vi "FitsCloseFile.vi"(8 "error in (no error)":errorcluster, 10 "ref in":u64, 11 "CFitsIO in":refnum<class "CFitsIO.lvclass">) -> (0 "error out":errorcluster, 1 "result":i32, 2 "ref out":u64, 3 "CFitsIO out":refnum<class "CFitsIO.lvclass">)   [LabVIEW 2016, in "CFitsIO.lvclass"]
uses:
  CFitsIO.lvclass
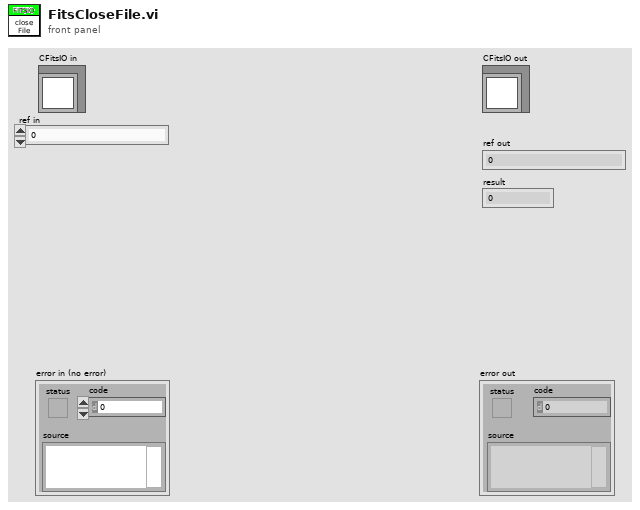
[diagram p1: front panel]
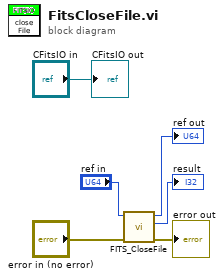
[diagram p0: block diagram]
diagram:
  n1 = call "FITS_CloseFile.vi"("error in"="error in (no error)", "ref in"="ref in") -> ("error out"=→"error out":errorcluster, "result"=→"result":i32, "ref out"=→"ref out":u64)  [unwired: 1 in, 6 out]
  "CFitsIO out" <- "CFitsIO in"
